vi "Measure 1D Array.vi"(0 "eye scan in":refnum<class "niHighSpeedSerial Eye Scan v1 Host.lvclass">, 5 "instance":u8, 7 "requested number of new points":i32, 9 "timeout (100 ms)":dbl=0.1, 11 "error in":errorcluster) -> (2 "timed out?":bool, 3 "retrieved number of new points":i32, 4 "eye scan out":refnum<class "niHighSpeedSerial Eye Scan v1 Host.lvclass">, 6 "bit error ratio per point":T3[](array[typedef]), 8 "error count per point":T1[](array[typedef]), 10 "sample count per point":T1[](array[typedef]), 14 "done?":bool, 15 "error out":errorcluster)   [LabVIEW 2014, in "niHighSpeedSerial Eye Scan v1 Host.lvclass"]
doc: "Returns the Bit Error Rate, sample count, and error count on points that have been measured in 1D arrays.\nThis VI returns under the following conditions, whichever comes first:\n1) The <b>requested number of new points</b> are completed on each channel.\n2) The <b>timeout</b> is reached.\n3) The last point of the scan finishes measuring on all channels.\n\n<B>Input Parameters</B>\n\n<B>eye scan in</B> Takes in a reference to your session from the previous VI.\n\n<B>instance</B> The instance of the channel to be used.\n\n<B>requested number of new points</B> The number of new points to return, assuming that timeout is not reached, the entire scan doesn't complete, and no errors occur.\n\n<B>timeout (100 ms)</B> The amount of time (in seconds) before timing timing out.\nSpecifying '-1' prevents 'timed out' from ever returning true.\n\n<B>error in</B> describes error conditions that occur before this node runs. This input provides standard 'error in' functionality.\n\n<B>Output Parameters</B>\n\n<B>retrieved number of new points</B> The number of new points that were retrieved in this call to Measure.\n\n<B>eye scan out</B> passes a reference to your session to the next VI.\n\n<B>bit error rate per point</B> is the calculated statistical bit error rate based on the number of error counts and sample counts received.\n\n<B>bit error rate per point.point offset</B> The vertical and horizontal point offsets\n\n<B>bit error rate per point.point offset.horizontal offset</B> The horizontal offset of the point.\n\n<B>bit error rate per point.point offset.vertical offset</B> The vertical offset of the point.\n\n<B>bit error rate per point.Bit Error Rate</B> is the measured statistical number of bit errors divided by the number of sample counts at a given point.\nNote that when DFE mode is selected, the bit error rate is the average of the positive and negative bit error rates.\n\n<B>error count per point</B> is the number of errors received at a given point.\n\n<B>error count per point.point offset</B> The vertical and horizontal point offsets\n\n<B>error count per point.point offset.horizontal offset</B> The horizontal offset of the point.\n\n<B>error count per point.point offset.vertical offset</B> The vertical offset of the point.\n\n<B>error count per point.count</B> is the number of errors received at a given point.\n\n<B>sample count per point</B> is the number of samples measured at a given point.\n\n<B>sample count per point.point offset</B> The vertical and horizontal point offsets\n\n<B>sample count per point.point offset.horizontal offset</B> The horizontal offset of the point.\n\n<B>sample count per point.point offset.vertical offset</B> The vertical offset of the point.\n\n<B>sample count per point.count</B> is the number of samples measured at a given point.\n\n<B>timed out?</B> returns true if at least 'timeout' amount of time has passed.\n\n<B>done?</B> returns true if the Eye Scan algorithm has completed measuring all points.\n\n<B>error out</B> contains error information. This output provides standard 'error out' functionality."
uses:
  <instrlib>/niHighSpeedSerial/Eye Scan/v1/Host/Eye Scan/niHighSpeedSerial Eye Scan v1 Host.lvclass
  <instrlib>/niHighSpeedSerial/Eye Scan/v1/Host/Eye Scan/Public/BER 1D.ctl
  <instrlib>/niHighSpeedSerial/Eye Scan/v1/Host/Common/Public/Point Offsets.ctl
  <instrlib>/niHighSpeedSerial/Eye Scan/v1/Host/Eye Scan/Public/Count 1D.ctl
  <instrlib>/niHighSpeedSerial/Eye Scan/v1/Host/Eye Scan/niHighSpeedSerial Eye Scan v1 Host.lvclass/niHighSpeedSerial Eye Scan v1 Host.ctl
  <instrlib>/niHighSpeedSerial/Eye Scan/v1/Host/Impl/Eye Scan Point Iterator/niHighSpeedSerial Eye Scan Point Iterator v1 Host.lvclass
  <instrlib>/niHighSpeedSerial/Eye Scan/v1/Host/Common/niHighSpeedSerial Eye Scan Common v1 Host.lvlib
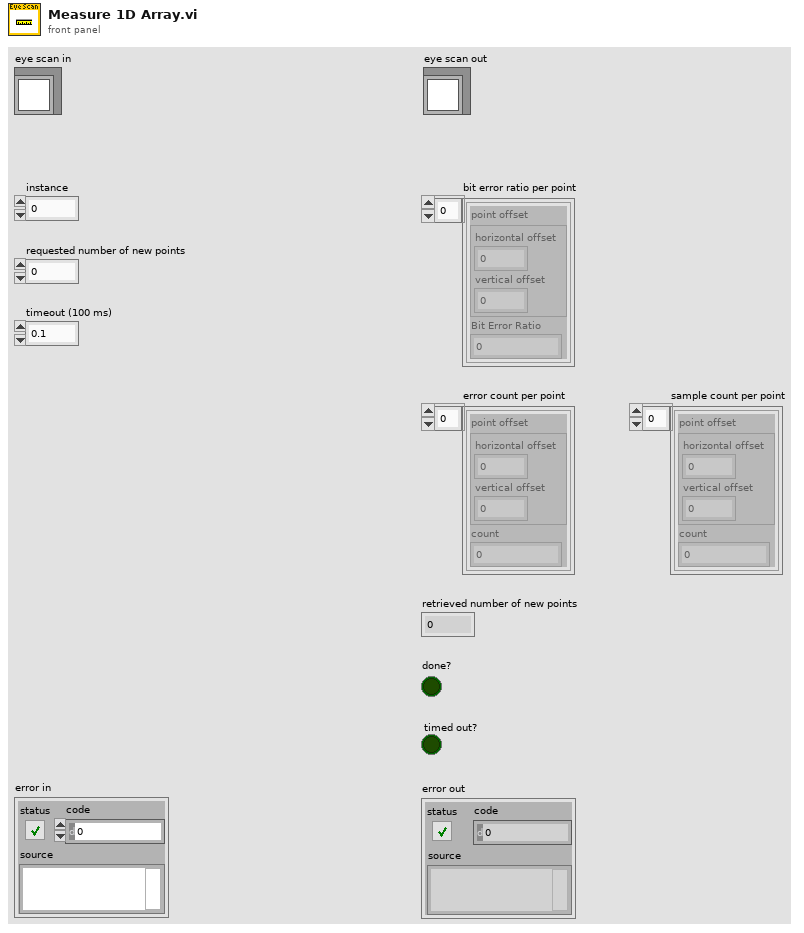
[diagram p1: front panel]
types:
  T1 = typedef "niHighSpeedSerial Eye Scan v1 Host.lvclass/Count 1D.ctl" = cluster{"point offset":T2, "count":u64}
  T2 = typedef "niHighSpeedSerial Eye Scan Common v1 Host.lvlib/Point Offsets.ctl" = cluster{"horizontal offset":i16, "vertical offset":i8}
  T3 = typedef "niHighSpeedSerial Eye Scan v1 Host.lvclass/BER 1D.ctl" = cluster{"point offset":T2, "Bit Error Ratio":dbl}
  T4 = typedef "niHighSpeedSerial Eye Scan v1 Host.lvclass/Private Data.ctl" = cluster{"instruction target":refnum<class "niInstr Instruction Target v1 Host.lvclass">, "channels":T5[], "measure state":T6, "rx output divider":T7, "equalization mode":T8, "rx data width":T9, "BER floor":dbl, "number of points completed":i32, "rx output divider configured?":bool, "equalization mode configured?":bool, "rx data width configured?":bool}
  T5 = typedef "niHighSpeedSerial Eye Scan v1 Host.lvclass/Channel Data.ctl" = cluster{"instance":u8, "channel":refnum<class "niHighSpeedSerial Eye Scan Single Point v1 Host.lvclass">, "point iterator":refnum<class "niHighSpeedSerial Eye Scan Point Iterator v1 Host.lvclass">}
  T6 = typedef "niHighSpeedSerial Eye Scan v1 Host.lvclass/Measure State.ctl" = enum16{"Uninitialized", "Initialized", "Ready", "Measuring", "Finished", "Aborted"}
  T7 = typedef "niHighSpeedSerial Eye Scan Common v1 Host.lvlib/RX Output Divider.ctl" = enum16{"1", "2", "4", "8", "16"}
  T8 = typedef "niHighSpeedSerial Eye Scan Common v1 Host.lvlib/Equalization Mode.ctl" = enum16{"DFE", "LPM"}
  T9 = typedef "niHighSpeedSerial Eye Scan Common v1 Host.lvlib/Data Width.ctl" = enum16{"16 Bit", "20 Bit", "32 Bit", "40 Bit"}
  T10 = typedef "niHighSpeedSerial Eye Scan Common v1 Host.lvlib/Point.ctl" = cluster{"point offsets":T2, "sample count":u64, "error count":u64, "bit error ratio":dbl}
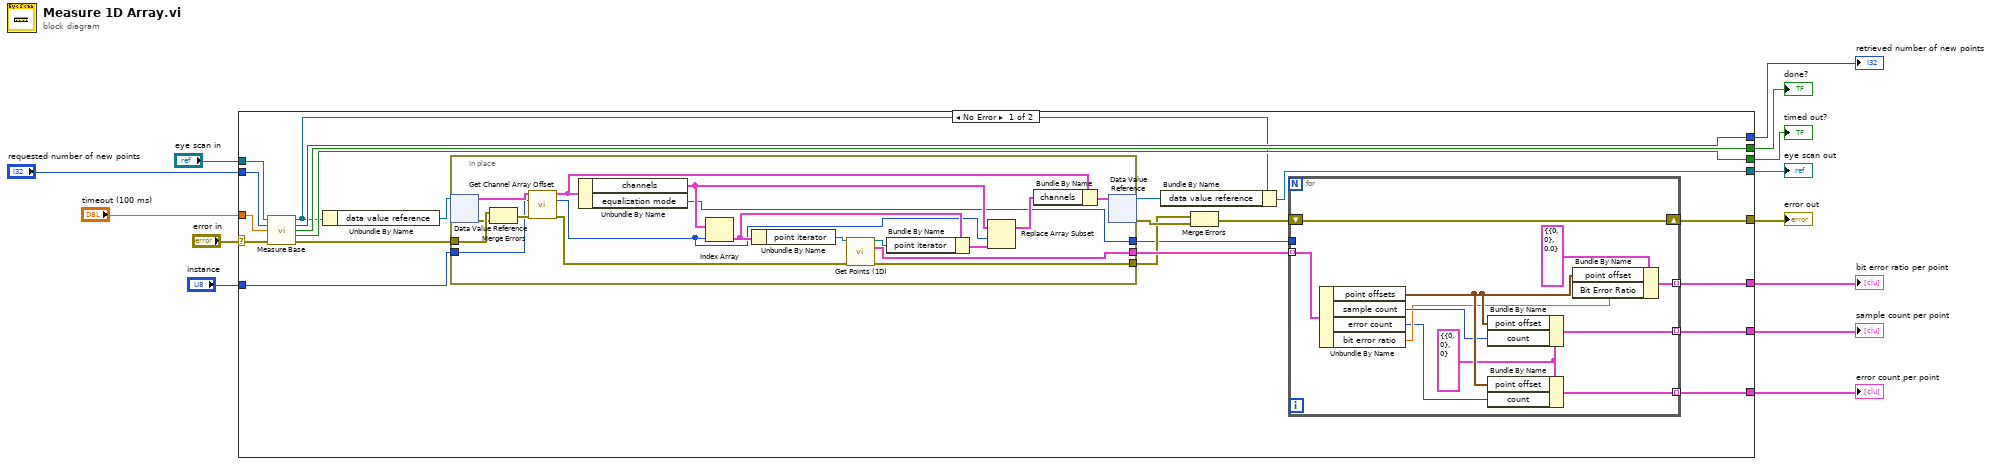
[diagram p0: block diagram]
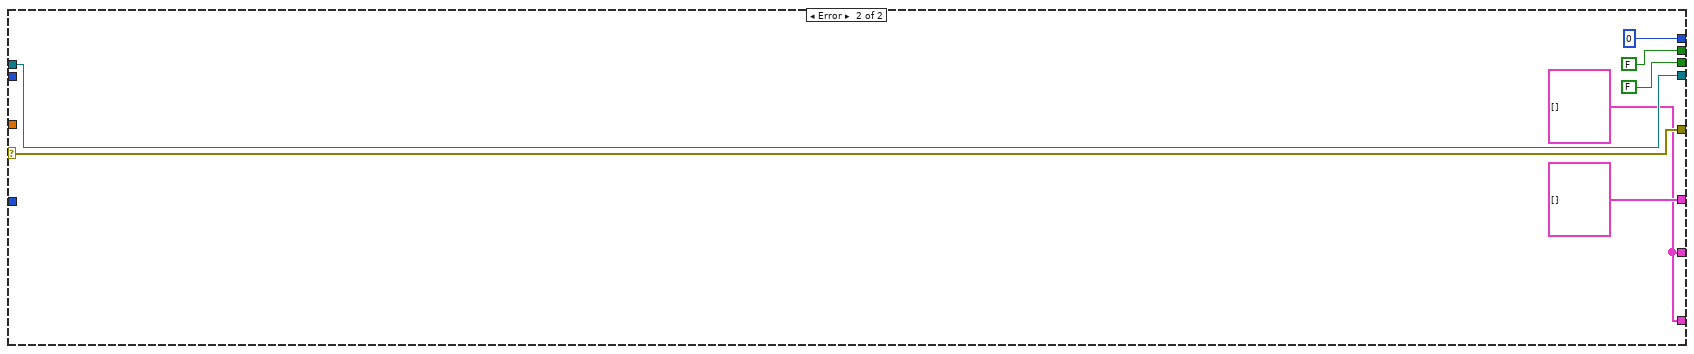
[diagram p2: hidden frame]
diagram:
  n1 = case shown="No Error" "error in" {
    selector: "error in" -> [w31 w71]
    tunnel: [w22 w71] -> w12
    tunnel: "requested number of new points" -> [w35 _]
    tunnel: "timeout (100 ms)" -> [w33 _]
    tunnel: [w19 w70] -> w9
    tunnel: "eye scan in" -> [w32 w70]
    tunnel: "instance" -> [w25 _]
    tunnel: [w27 w67] -> w6
    tunnel: [w30 FALSE ("Done?")] -> w5
    tunnel: [w34 0 ("Retrieved Number of New Points")] -> w4
    tunnel: [w29 T3[] []] -> w3
    tunnel: [w28 w67] -> w2
    tunnel: [w23 FALSE ("Timed Out?")] -> w1
    frame No Error {
      n2 = call <instrlib>:"Measure Base.vi"("eye scan in"=w32, "requested number of new points"=w35, "timeout (100 ms)"=w33, "error in"=w31) -> ("eye scan out"=w18:refnum<class "niHighSpeedSerial Eye Scan v1 Host.lvclass">, "retrieved number of new points"=w34:i32, "last point measured?"=w30:bool, "timed out?"=w23:bool, "error out"=w24:errorcluster)  [unwired: 7 in]
      n3 = Unbundle By Name(w18) -> ("data value reference"=w26:refnum<data-value>)
      n4 = in-place {
        in-place-border: w25 -> [w40]
        in-place-border: w24 -> [w53]
        in-place-border: [w50] -> w17
        in-place-border: [w38] -> w15
        in-place-border: [w36] -> w14
        n5 = in-place-dvr #1(w26) -> (w42:T4, w52:errorcluster)
        n6 = Merge Errors(w53, w52) -> (w43:errorcluster)
        n7 = call <instrlib>:"Get Channel Array Offset.vi"("private data"=w42, "instance"=w40, "error in"=w43) -> ("private data out"=w41:T4, "channel array offset"=w37:i32, "error out"=w39:errorcluster)  [unwired: 10 in]
        n8 = Unbundle By Name(w41) -> ("channels"=w47:T5[], "equalization mode"=w36:T8)
        n9 = Index Array(array=w47, index=w37) -> (element=w49:T5)
        n10 = Unbundle By Name(w49) -> ("point iterator"=w51:refnum<class "niHighSpeedSerial Eye Scan Point Iterator v1 Host.lvclass">)
        n11 = call-dynamic "Get Points (1D).vi"("eye scan point iterator"=w51, "error in"=w39) -> ("eye scan point iterator out"=w48:refnum<class "niHighSpeedSerial Eye Scan Point Iterator v1 Host.lvclass">, "array of points"=w50:T10[], "error out"=w38:errorcluster)  [unwired: 11 in]
        n12 = Bundle By Name(cluster=w49, "point iterator"=w48) -> (w46:T5)
        n13 = Replace Array Subset(array=w47, new element=w46, index=w37) -> (w45:T5[])
        n14 = Bundle By Name(cluster=w41, "channels"=w45) -> (w44:T4)
        n15 = in-place-dvr #1(w44) -> (w20:refnum<data-value>, w16:errorcluster)
      }
      n16 = Bundle By Name(cluster=w18, "data value reference"=w20) -> (w19:refnum<class "niHighSpeedSerial Eye Scan v1 Host.lvclass">)
      n17 = Merge Errors(w15, w16) -> (w21:errorcluster)
      n18 = for {
        tunnel: [w63] -> w29 mode=indexing
        tunnel: [w62] -> w28 mode=indexing
        tunnel: [w59] -> w27 mode=indexing
        shift-right: [w57] -> w22
        shift-left: w21 -> [w57]
        tunnel: w17 -> [w58] mode=indexing
        tunnel: w14 -> [_]
        w60 = T1 {"point offset"={"horizontal offset"=0, "vertical offset"=0}, "count"=0} ("Count 1D")
        n19 = Unbundle By Name(w58) -> ("point offsets"=w61:T2, "sample count"=w56:u64, "error count"=w54:u64, "bit error ratio"=w55:dbl)
        n20 = Bundle By Name(cluster=w60, "point offset"=w61, "count"=w56) -> (w62:T1)
        n21 = Bundle By Name(cluster=w60, "point offset"=w61, "count"=w54) -> (w59:T1)
        n22 = Bundle By Name(cluster=T3 {"point offset"={"horizontal offset"=0, "vertical offset"=0}, "Bit Error Ratio"=0.0} ("BER 1D"), "point offset"=w61, "Bit Error Ratio"=w55) -> (w63:T3)
      }
    }
    frame Error {
      w67 = T1[] []
    }
  }
  "error out" <- w12
  "eye scan out" <- w9
  "bit error ratio per point" <- w3
  "error count per point" <- w6
  "sample count per point" <- w2
  "done?" <- w5
  "retrieved number of new points" <- w4
  "timed out?" <- w1
